vi "Run_important_tasks.vi"(7 "pulses previous":i64, 8 "error in (no error)":errorcluster, 9 "ControlQueue":refnum<queue>, 10 "divider":i8=10, 11 "DAQmxTaksContainer_General in":refnum<class "DAQmxTaksContainer_General.lvclass">) -> (0 "error out":errorcluster, 2 "pulses":i64, 3 "DAQmxTaksContainer_General out":refnum<class "DAQmxTaksContainer_General.lvclass">)   [LabVIEW 2020, in "DAQmxTaksContainer_General.lvclass"]
uses:
  DAQmxTaksContainer_General.lvclass
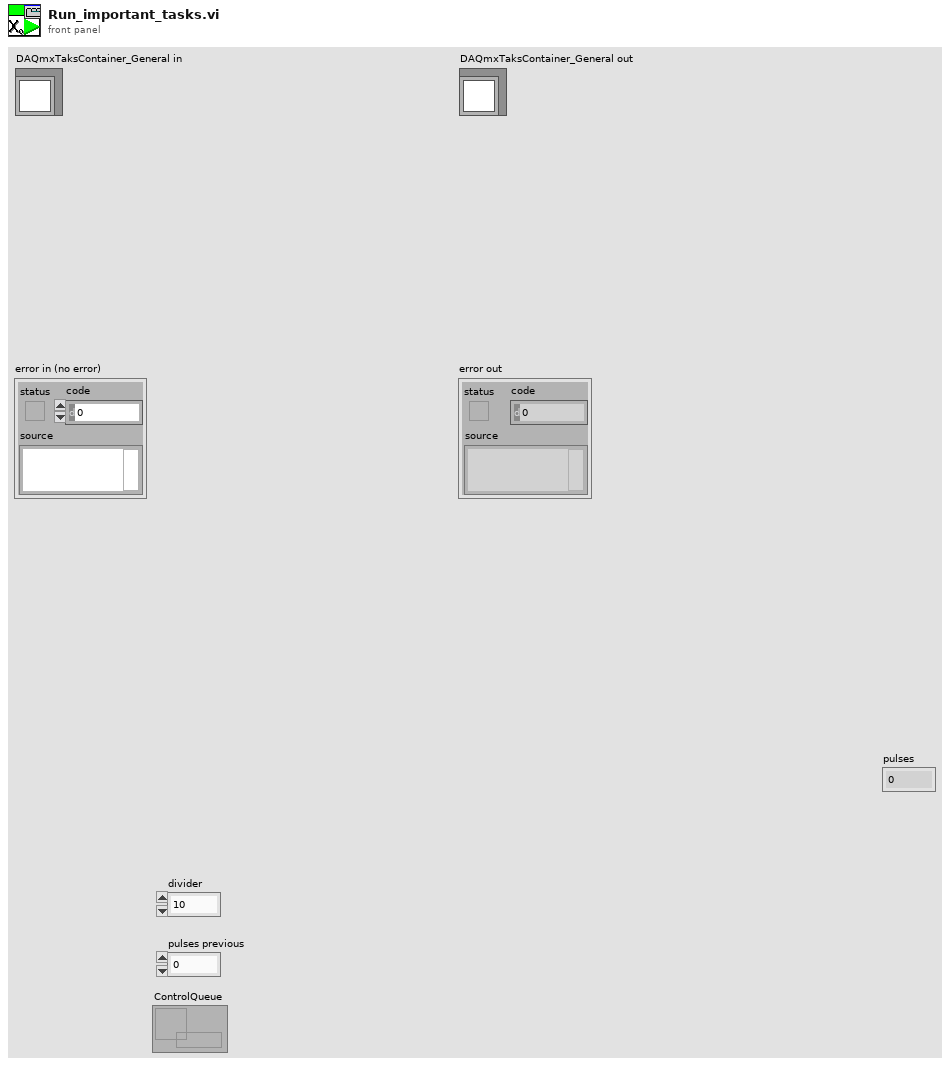
[diagram p1: front panel]
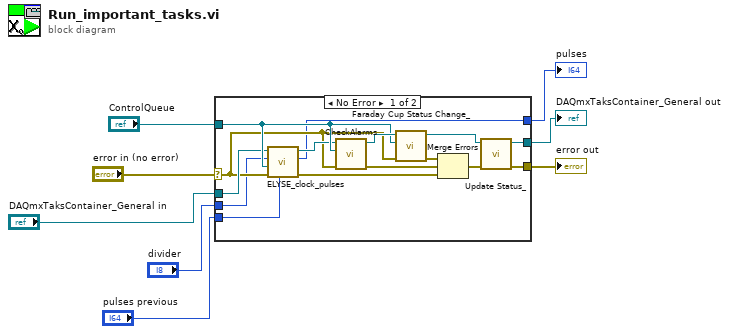
[diagram p0: block diagram]
diagram:
  n1 = case shown="No Error" "error in (no error)" {
    selector: "error in (no error)" -> [w13 w26]
    tunnel: [w17 w26] -> w2
    tunnel: [w21 w25] -> w1
    tunnel: "DAQmxTaksContainer_General in" -> [w15 w25]
    tunnel: "divider" -> [w11 _]
    tunnel: "ControlQueue" -> [w16 _]
    tunnel: "pulses previous" -> [w10 w24]
    tunnel: [w9 w24] -> w5
    frame No Error {
      n2 = call "ELYSE_clock_pulses.vi"("pulses previous"=w10, "error in (no error)"=w13, "ControlQueue"=w16, "divider"=w11, "DAQmxTaksContainer_General in"=w15) -> ("error out"=w12:errorcluster, "pulses"=w9:i64, "DAQmxTaksContainer_General out"=w14:refnum<class "DAQmxTaksContainer_General.lvclass">)  [unwired: 4 in]
      n3 = call "CheckAlarms.vi"("error in (no error)"=w13, "ControlQueue"=w16, "DAQmxTaksContainer_General in"=w14) -> ("error out"=w23:errorcluster, "DAQmxTaksContainer_General out"=w20:refnum<class "DAQmxTaksContainer_General.lvclass">)  [unwired: 7 in]
      n4 = call "Faraday Cup Status Change_.vi"("error in (no error)"=w13, "ControlQueue"=w16, "DAQmxTaksContainer_General in"=w20) -> ("error out"=w19:errorcluster, "DAQmxTaksContainer_General out"=w18:refnum<class "DAQmxTaksContainer_General.lvclass">)  [unwired: 7 in]
      n5 = Merge Errors(w19, w23, w12) -> (w22:errorcluster)
      n6 = call "Update Status_.vi"("error in (no error)"=w22, "DAQmxTaksContainer_General in"=w18) -> ("error out"=w17:errorcluster, "DAQmxTaksContainer_General out"=w21:refnum<class "DAQmxTaksContainer_General.lvclass">)  [unwired: 8 in]
    }
    frame Error {
    }
  }
  "error out" <- w2
  "DAQmxTaksContainer_General out" <- w1
  "pulses" <- w5
